vi "Init.vi"(8 "error in (no error)":errorcluster, 11 "Data in":refnum<class "Multi_Bus.lvclass">) -> (0 "error out":errorcluster, 3 "Data out":refnum<class "Multi_Bus.lvclass">)   [LabVIEW 2021, in "Multi_Bus.lvclass"]
uses:
  Multi_Bus.lvclass
  <vilib>/TSA/Abstract Data Classes/Abs_Types/Type/Abs_Type.lvclass
  Multi_Bus.lvclass/Multi_Bus.ctl
  Bus_Access/Bus_Access.lvclass/Bus_Access.ctl
  <vilib>/TSA/Abstract Data Classes/Abs_Types/Type/Abs_Type.lvclass/Abs_Type.ctl
  <vilib>/Utility/error.llb/DialogType.ctl
  <vilib>/TSA/Abstract Data Classes/Abs_Types/Type/Properties/Write Var_Index.vi
  Bus_Access/Properties/Read Vars.vi
  Bus_Access/Properties/Read Tag Root.vi
  Bus_Access/Properties/Read Tags.vi
  Properties/Read Var Access.vi
  Properties/Write Var Access.vi
  Properties/Write Var Map.vi
  Bus_Access/Bus_Access.lvclass
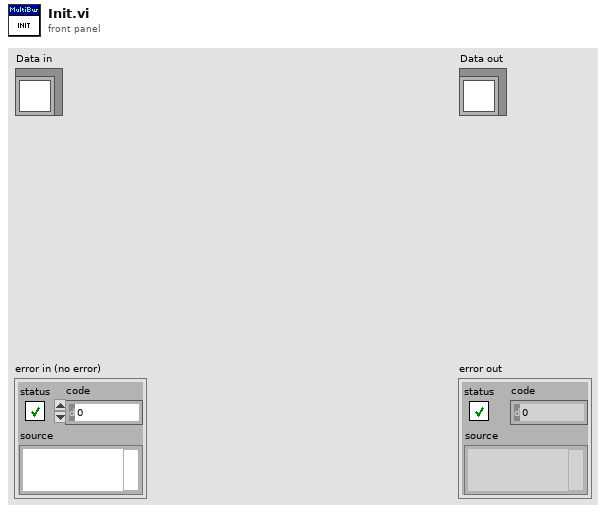
[diagram p1: front panel]
types:
  T1 = typedef "DialogType.ctl" = u16
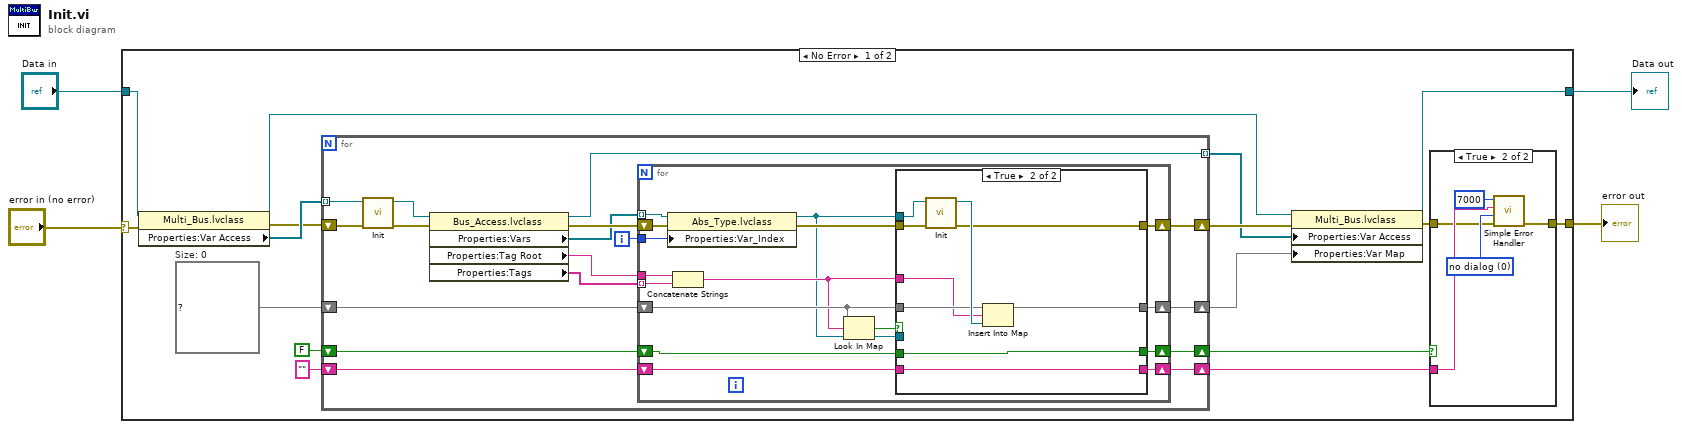
[diagram p0: block diagram]
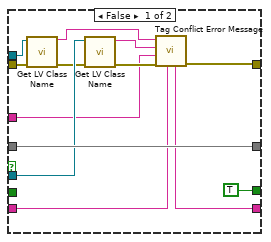
[diagram p3: hidden frame]
diagram:
  n1 = case shown="No Error" "error in (no error)" {
    selector: "error in (no error)" -> [w20 w83]
    tunnel: "Data in" -> [w19 w84]
    tunnel: [w6 w83] -> w2
    tunnel: [w13 w84] -> w1
    frame No Error {
      w12 = map{string, refnum<class "Abs_Type.lvclass">} {}  # Size: 0
      n2 = property class="Multi_Bus.lvclass"(reference=w19, error in=w20) -> (reference out=w14:refnum<class "Multi_Bus.lvclass">, error out=w17:errorcluster, "Properties:Var Access"=w18:refnum<class "Bus_Access.lvclass">[])
      n3 = for {
        tunnel: w18 -> [w42] mode=indexing
        shift-right: [w32] -> w16
        shift-left: w17 -> [w43]
        tunnel: [w39] -> w15 mode=indexing
        shift-right: [w36] -> w11
        shift-left: w12 -> [w35]
        shift-right: [w31] -> w5
        shift-left: "" -> [w30]
        shift-right: [w29] -> w8
        shift-left: FALSE -> [w28]
        i -> [w33]
        n4 = call-dynamic "Init.vi"("error in (no error)"=w43, "Data in"=w42) -> ("error out"=w41:errorcluster, "Data out"=w40:refnum<class "Bus_Access.lvclass">)  [unwired: 8 in]
        n5 = property class="Bus_Access.lvclass"(reference=w40, error in=w41) -> (reference out=w39:refnum<class "Bus_Access.lvclass">, error out=w34:errorcluster, "Properties:Vars"=w27:refnum<class "Abs_Type.lvclass">[], "Properties:Tag Root"=w38:string, "Properties:Tags"=w37:string[])
        n6 = for {
          tunnel: w38 -> [w60]
          tunnel: w37 -> [w59] mode=indexing
          shift-right: [w58] -> w36
          shift-left: w35 -> [w54]
          tunnel: w33 -> [w56]
          shift-right: [w51] -> w32
          shift-left: w34 -> [w57]
          shift-right: [w48] -> w31
          shift-left: w30 -> [w47]
          shift-right: [w46] -> w29
          shift-left: w28 -> [w45]
          tunnel: w27 -> [w44] mode=indexing
          n7 = property class="Abs_Type.lvclass"(reference=w44, error in=w57, "Properties:Var_Index"=w56) -> (reference out=w52:refnum<class "Abs_Type.lvclass">, error out=w55:errorcluster)
          n8 = Concatenate Strings(w60, w59) -> (w53:string)
          n9 = Look In Map(map=w54, key=w53, default value=w52) -> (key not found?=w50:bool, value=w49:refnum<class "Abs_Type.lvclass">)
          n10 = case shown="True" w50 {
            tunnel: [w73 w82] -> w58
            tunnel: w55 -> [w71 w81]
            tunnel: w54 -> [w73 w79]
            tunnel: w53 -> [w64 w78]
            tunnel: w52 -> [w70 w77]
            tunnel: [w67 w76] -> w51
            tunnel: w49 -> [w72 _]
            tunnel: [w63 w75] -> w48
            tunnel: w47 -> [w62 w75]
            tunnel: [TRUE w74] -> w46
            tunnel: w45 -> [_ w74]
            frame False {
              n11 = call <vilib>:"Get LV Class Name.vi"("error in (no error)"=w71, "object"=w70) -> ("error out"=w69:errorcluster, "class name"=w66:string)  [unwired: 8 in]
              n12 = call <vilib>:"Get LV Class Name.vi"("error in (no error)"=w69, "object"=w72) -> ("error out"=w68:errorcluster, "class name"=w65:string)  [unwired: 8 in]
              n13 = call "Tag Conflict Error Message.vi"("Previous Error Message"=w62, "error in (no error)"=w68, "Tag Name"=w64, "Conflict Class"=w65, "Original Class"=w66) -> ("error out"=w67:errorcluster, "Error Message"=w63:string)  [unwired: 5 in]
            }
            frame True {
              n14 = call-dynamic "Init.vi"("error in (no error)"=w81, "Data in"=w77) -> ("error out"=w76:errorcluster, "Data out"=w80:refnum<class "Abs_Type.lvclass">)  [unwired: 8 in]
              n15 = Insert Into Map(map in=w79, key=w78, value=w80) -> (map out=w82:map{string, refnum<class "Abs_Type.lvclass">})  [unwired: 2 out]
            }
          }
        }
      }
      n16 = property class="Multi_Bus.lvclass"(reference=w14, error in=w16, "Properties:Var Access"=w15, "Properties:Var Map"=w11) -> (reference out=w13:refnum<class "Multi_Bus.lvclass">, error out=w7:errorcluster)
      n17 = case shown="True" w8 {
        tunnel: w7 -> [w21 w22]
        tunnel: [w21 w26] -> w6
        tunnel: w5 -> [_ w23]
        frame False {
        }
        frame True {
          w25 = T1 0 items=["no dialog", "OK message", "continue or stop message", "OK message + warnings", "continue/stop + warnings"] ("type of dialog (OK msg:1)")
          n18 = call <vilib>:"Simple Error Handler.vi"("error code (no error:0)"=7000, "error source (\" \")"=w23, "type of dialog (OK msg:1)"=w25, "error in (no error)"=w22) -> ("error out"=w26:errorcluster)  [unwired: 1 in, 4 out]
        }
      }
    }
    frame Error {
    }
  }
  "error out" <- w2
  "Data out" <- w1
